vi "Intrumento_1.vi"() -> ()   [LabVIEW 2016]
uses:
  Global_1.vi
  Global_2.vi
panel:
  out "Numeric Control_2":dbl
  out "Boolean_2":bool
  in  "Numeric Control_1":dbl
  in  "Boolean_1":bool
  in  "Stop Button":bool
  out "Usuario 2":string
  in  "Usuario 1":string
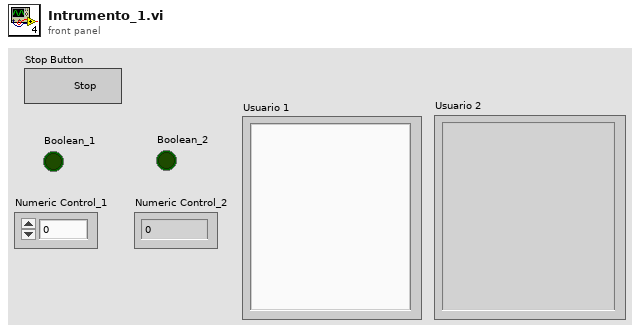
[diagram p1: front panel]
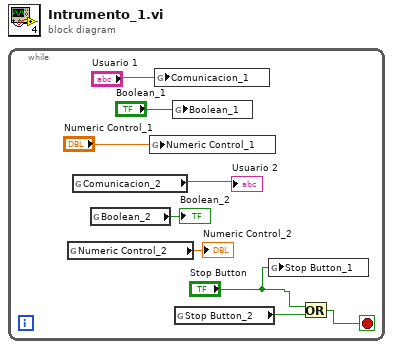
[diagram p0: block diagram]
diagram:
  n1 = while {
    stop <- w2 stop-if-true
    n2 = global read "Global_2.vi" "Numeric Control_2"() -> (→"Numeric Control_2":dbl)
    n3 = global read "Global_2.vi" "Comunicacion_2"() -> (→"Usuario 2":string)
    n4 = global read "Global_2.vi" "Boolean_2"() -> (→"Boolean_2":bool)
    n5 = global write "Global_1.vi" "Numeric Control_1"("Numeric Control_1") -> ()
    n6 = global write "Global_1.vi" "Comunicacion_1"("Usuario 1") -> ()
    n7 = global write "Global_1.vi" "Boolean_1"("Boolean_1") -> ()
    n8 = global read "Global_2.vi" "Stop Button_2"() -> (w3:bool)
    n9 = global write "Global_1.vi" "Stop Button_1"("Stop Button") -> ()
    n10 = Or(x="Stop Button", y=w3) -> (x .or. y?=w2:bool)
  }
